vi "capex profile.vi"() -> ()   [LabVIEW 2013]
panel:
  out "Current time":timestamp format="%<%X\n%x>T"
  out "Profile line":dbl
  in  "Stop Profile":bool
  out "profile times":timestamp[](array[timestamp])
  out "profile big chamber temp":dbl[](array[numeric]) format="%.2f"
  out "profile big chamber ramp":dbl[](array[numeric]) format="%.2f"
  out "profile chiller speed":string[](array[string])
  out "profile relay 4":string[](array[string])
  out "profile relay 3":string[](array[string])
  out "profile relay 2":string[](array[string])
  out "profile relay 1":string[](array[string])
  out "profile elapsed time":dbl[](array[numeric]) format="%.2f"
  out "profile AC volts":dbl[](array[numeric]) format="%.2f"
  out "profile AC current limit":dbl[](array[numeric]) format="%.2f"
  out "profile DC volts":dbl[](array[numeric]) format="%.2f"
  out "profile DC current limit":dbl[](array[numeric]) format="%.2f"
  out "profile little chamber temp":dbl[](array[numeric]) format="%.2f"
  out "profile little chamber ramp":dbl[](array[numeric]) format="%.2f"
  out "profile chiller temp":dbl[](array[numeric]) format="%.2f"
  in  "stop":bool
  in  "operation (0:open)":T1(ring)=enum."open or create"
  in  "make template":bool
  out "Profile running":bool
  out "Start time of last executed profile":timestamp
  out "Profile last executed":path
  in  "Loop profile when complete":bool
  in  "Execute profile":bool
  in  "Start in the future":bool
  out "Loaded profile":cluster{timestamp[], dbl[]}[](graph)
  in  "Load Profile":path
  in  "Scheduled start time":timestamp
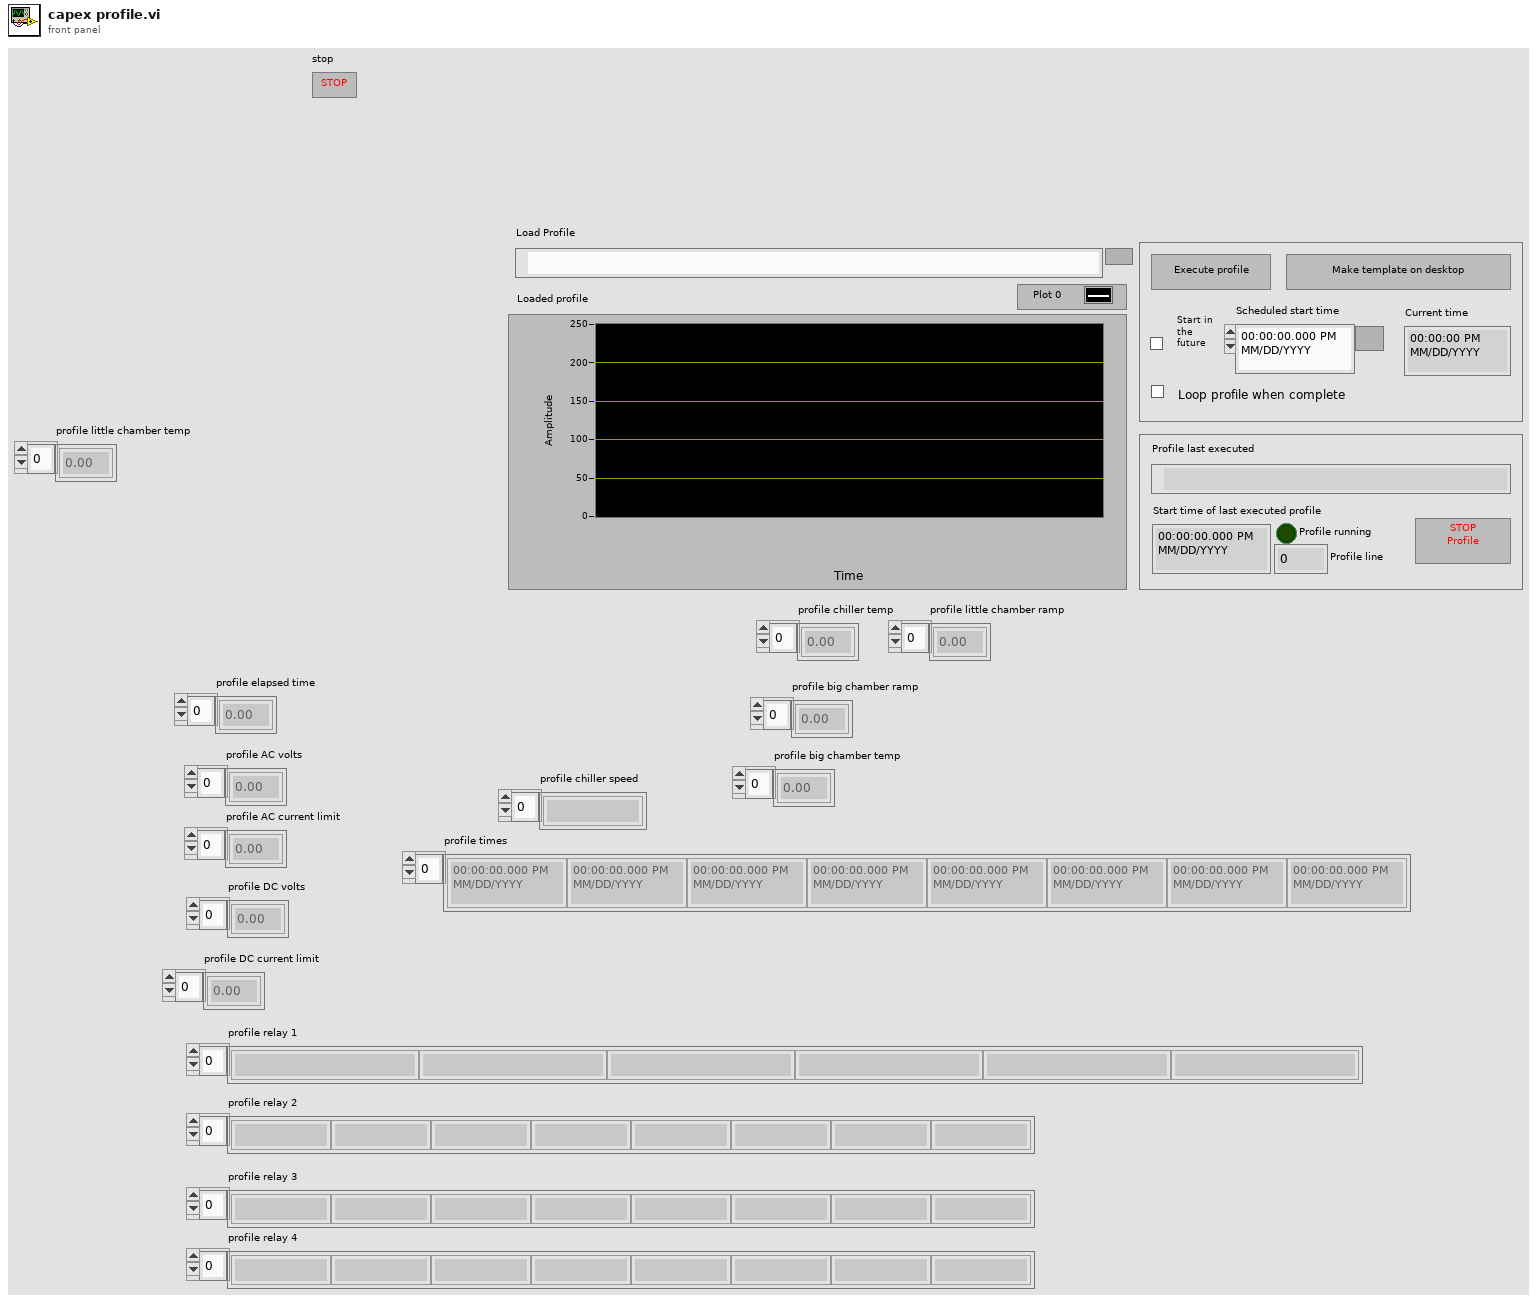
[diagram p1: front panel]
types:
  T1 = enum16{"open", "replace", "create", "open or create", "replace or create", "replace or create with confirmation"}
  T2 = enum8{"Enabled", "Disabled", "Disabled and Grayed Out"}
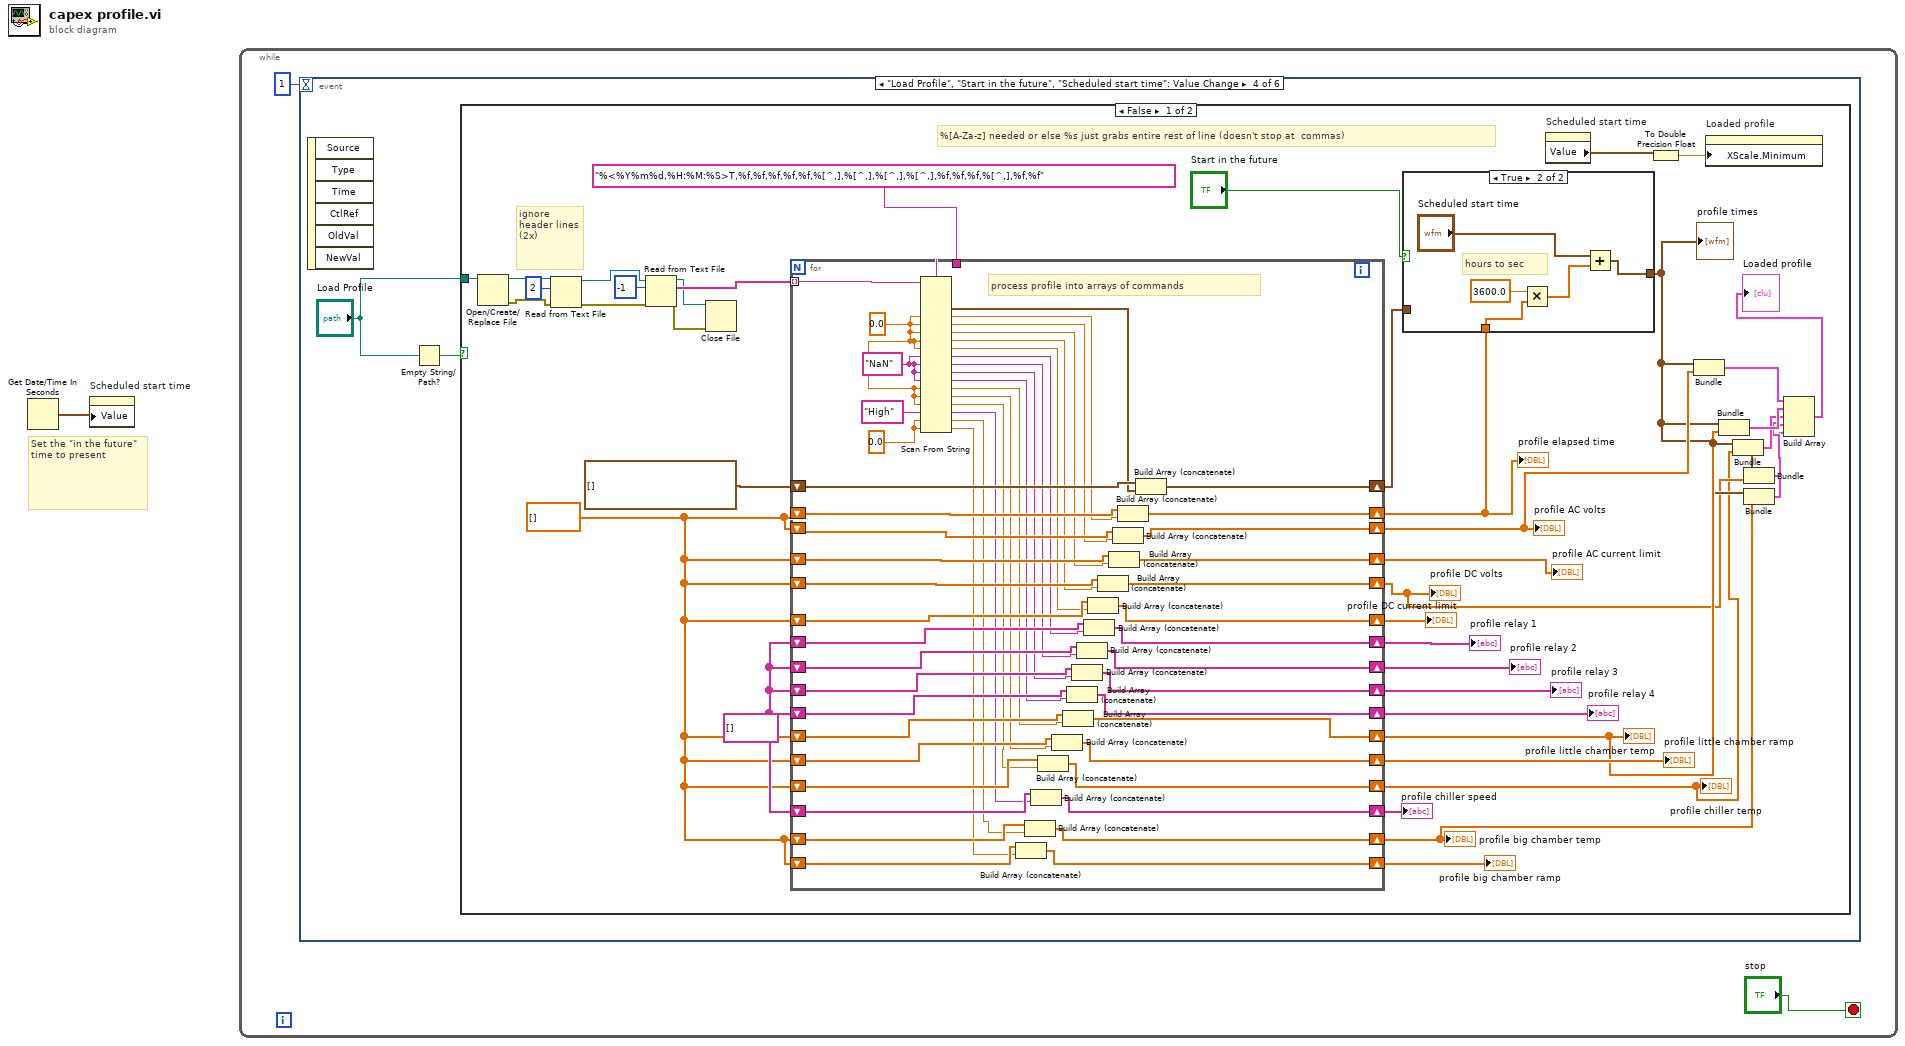
[diagram p0: block diagram]
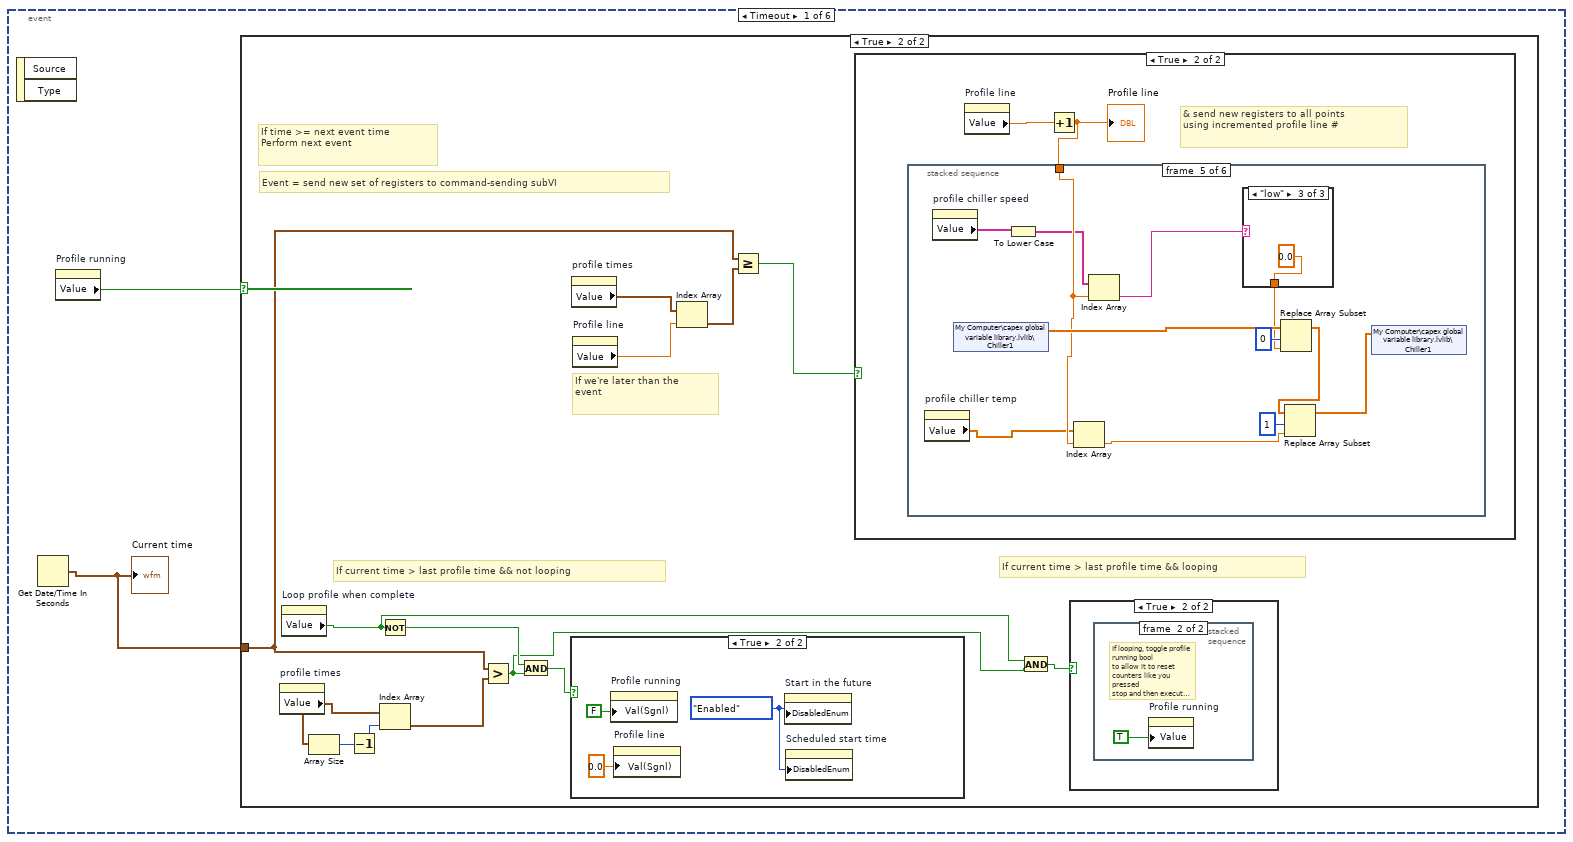
[diagram p2: hidden frame]
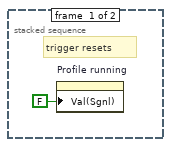
[diagram p5: hidden frame]
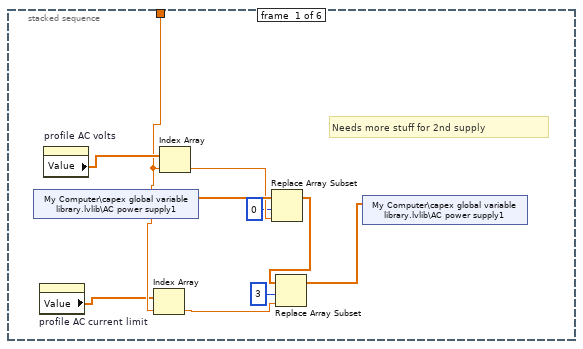
[diagram p7: hidden frame]
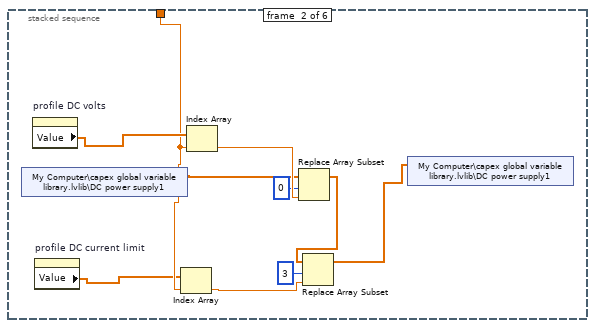
[diagram p8: hidden frame]
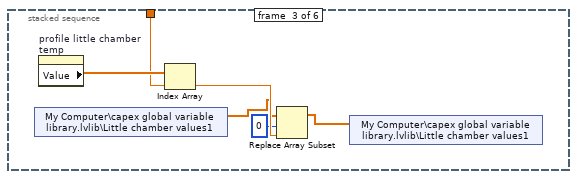
[diagram p9: hidden frame]
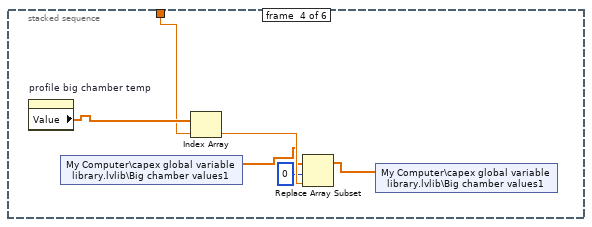
[diagram p10: hidden frame]
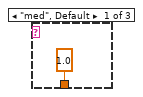
[diagram p11: hidden frame]
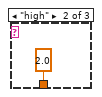
[diagram p12: hidden frame]
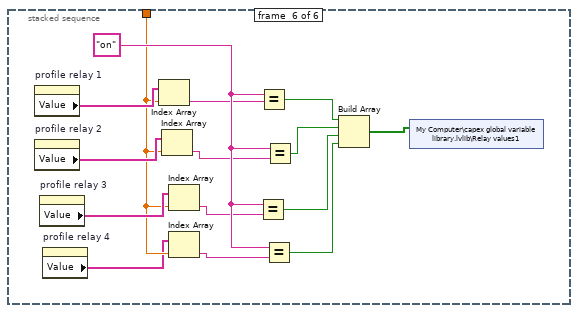
[diagram p13: hidden frame]
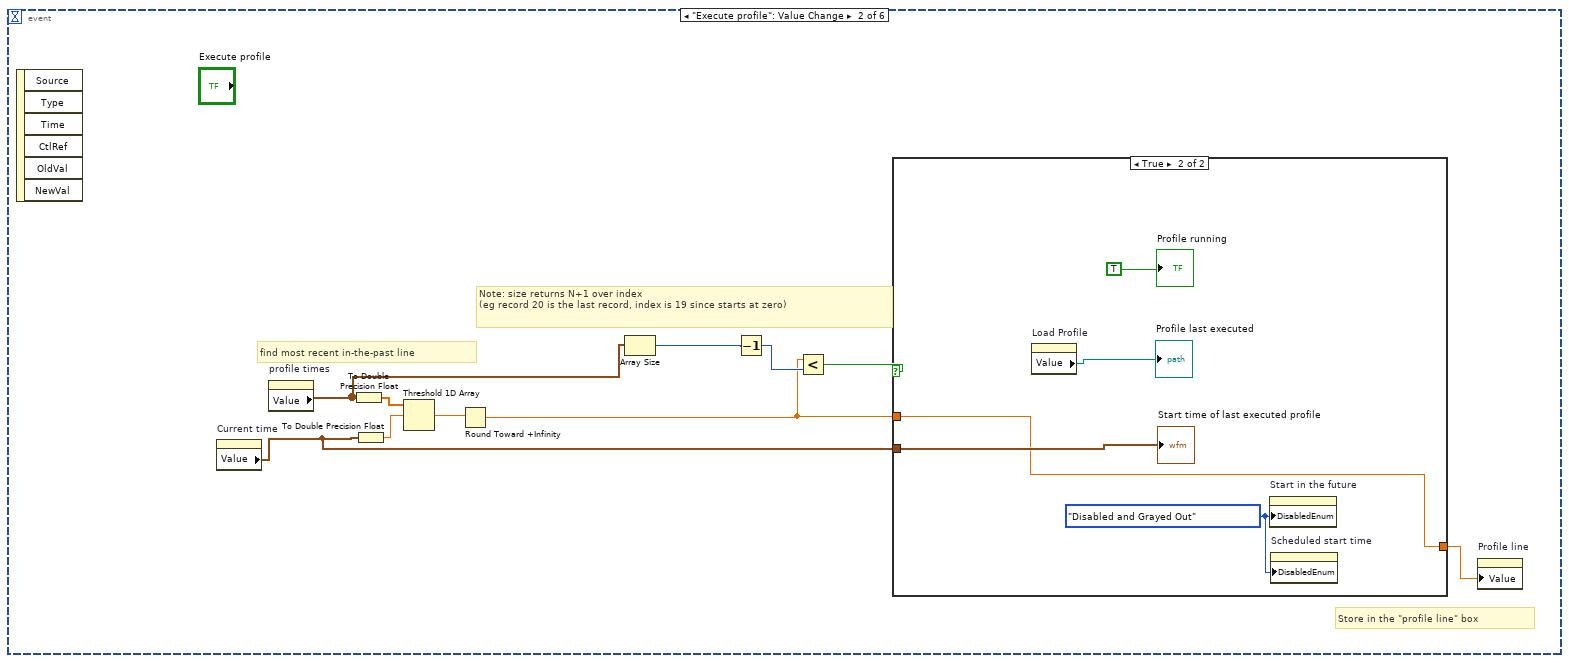
[diagram p15: hidden frame]
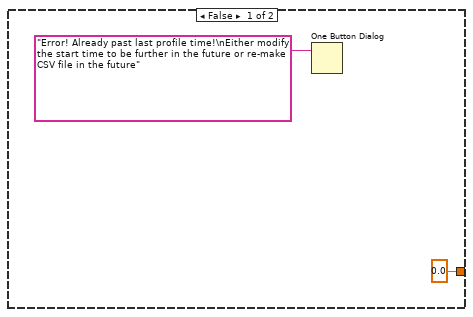
[diagram p16: hidden frame]
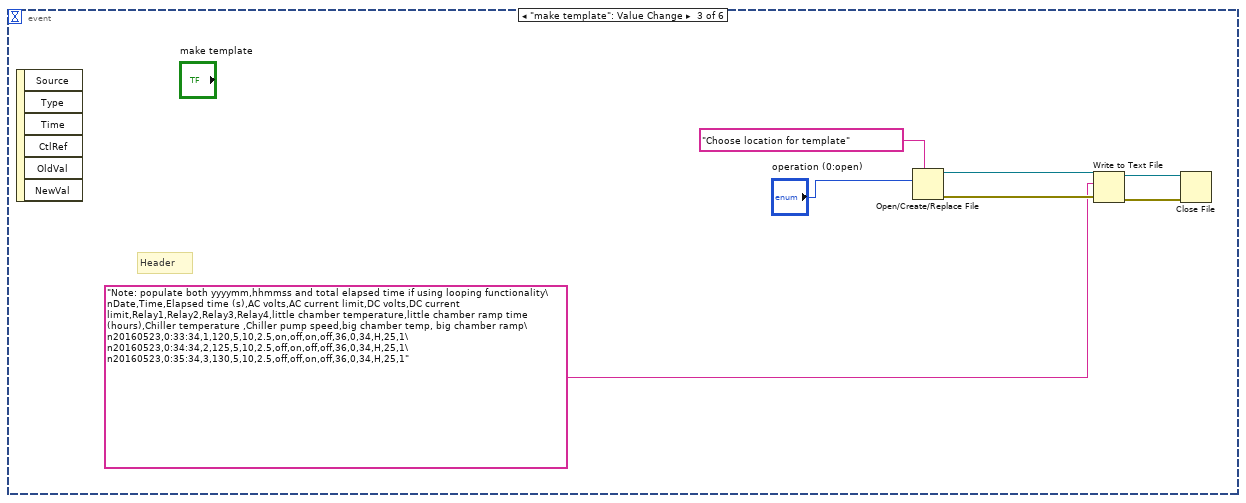
[diagram p17: hidden frame]
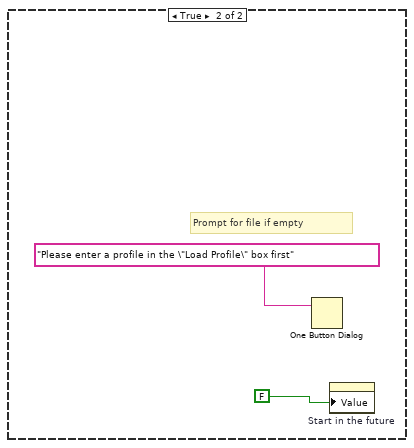
[diagram p19: hidden frame]
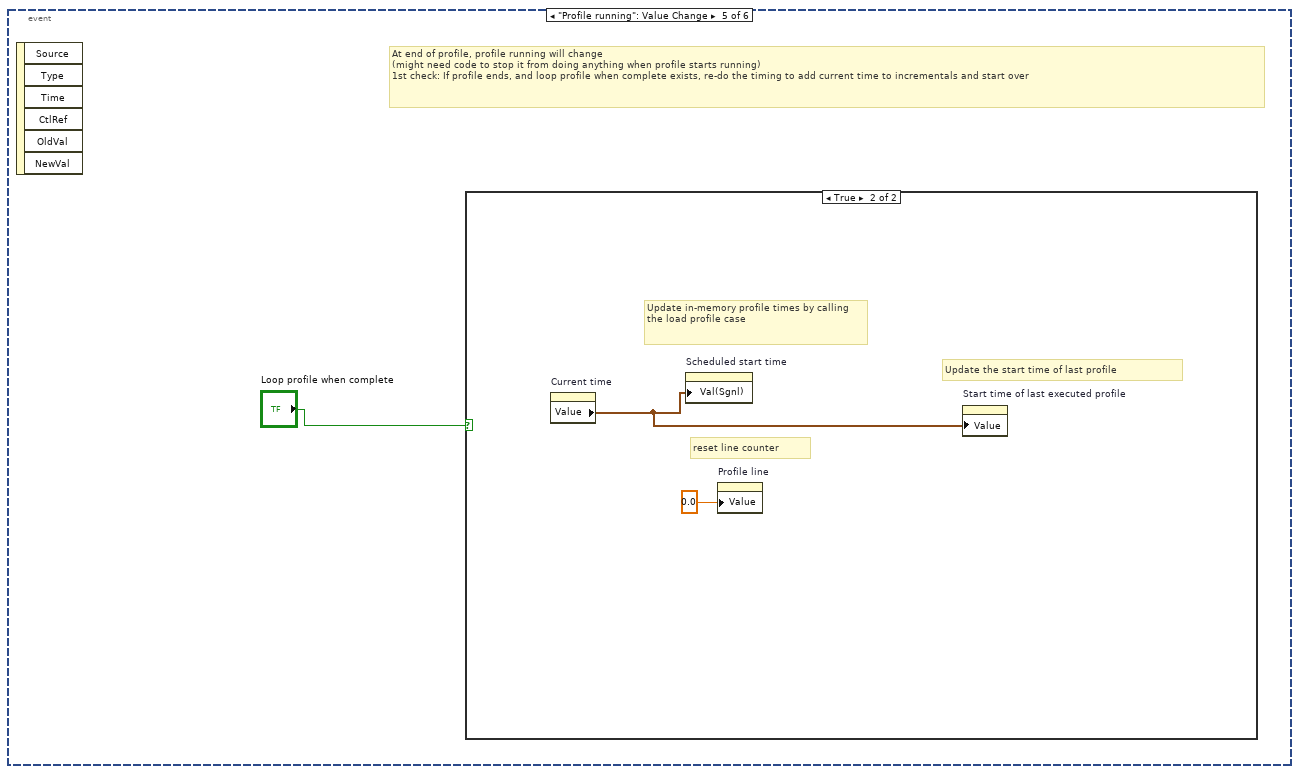
[diagram p20: hidden frame]
diagram:
  # "Set the \"in the future\" time to present"
  n1 = Get Date/Time In Seconds() -> (seconds since 1Jan1904=w1:timestamp)
  n2 = property on="Scheduled start time" class="AbsTime (strict)"("Value"=w1) -> ()  [unwired: 2 in, 2 out]
  n3 = while {
    stop <- "stop" stop-if-true
    n4 = event shown="[3] \"Load Profile\", \"Start in the future\", \"Scheduled start time\": Value Change" {
      selector: _ -> [_ _ _ _ _ _]
      dyn-events: _ -> [_ _ _ _ _ _]
      timeout: 1 -> [_ _ _ _ _ _]
      event Timeout {
        n5 = event-data() -> ()  [unwired: 1 in, 2 out]
        n6 = Get Date/Time In Seconds() -> (seconds since 1Jan1904=w4:timestamp)
        "Current time" <- w4
        n7 = property on="Profile running" class="Bool (strict)"() -> ("Value"=w5:bool)  [unwired: 2 in, 2 out]
        n8 = case shown="True" w5 {
          tunnel: w4 -> [_ w6]
          frame False {
          }
          frame True {
            # "If current time > last profile time && looping"
            # "If we're later than the\nevent"
            # "If current time > last profile time && not looping"
            # "Event = send new set of registers to command-sending subVI"
            # "If time >= next event time\nPerform next event"
            n9 = property on="profile times" class="Arr (strict)"() -> ("Value"=w17:timestamp[])  [unwired: 2 in, 2 out]
            n10 = property on="Loop profile when complete" class="Bool (strict)"() -> ("Value"=w8:bool)  [unwired: 2 in, 2 out]
            n11 = Array Size(array=w17) -> (size(s)=w19:i32)
            n12 = Decrement(x=w19) -> (x-1=w18:i32)
            n13 = Not(x=w8) -> (.not. x?=w14:bool)
            n14 = Index Array(array=w17, index=w18) -> (element=w16:timestamp)
            n15 = Greater?(x=w6, y=w16) -> (0:w7:bool)
            n16 = And(x=w14, y=w7) -> (x .and. y?=w15:bool)
            n17 = case shown="True" w15 {
              frame False {
              }
              frame True {
                w86 = T2."Enabled" ("Disabled")
                n18 = property on="Profile running" class="Bool (strict)"("Val(Sgnl)"=FALSE ("Value (Signaling)")) -> ()  [unwired: 2 in, 2 out]
                n19 = property on="Profile line" class="DigNum (strict)"("Val(Sgnl)"=0.0 ("Value (Signaling)")) -> ()  [unwired: 2 in, 2 out]
                n20 = property on="Start in the future" class="Bool (strict)"("DisabledEnum"=w86) -> ()  [unwired: 2 in, 2 out]
                n21 = property on="Scheduled start time" class="AbsTime (strict)"("DisabledEnum"=w86) -> ()  [unwired: 2 in, 2 out]
              }
            }
            n22 = property on="profile times" class="Arr (strict)"() -> ("Value"=w13:timestamp[])  [unwired: 2 in, 2 out]
            n23 = property on="Profile line" class="DigNum (strict)"() -> ("Value"=w12:dbl)  [unwired: 2 in, 2 out]
            n24 = Index Array(array=w13, index=w12) -> (element=w11:timestamp)
            n25 = Greater Or Equal?(x=w6, y=w11) -> (x >= y?=w10:bool)
            n26 = case shown="True" w10 {
              frame False {
              }
              frame True {
                # "& send new registers to all points\nusing incremented profile line #"
                n27 = property on="Profile line" class="DigNum (strict)"() -> ("Value"=w23:dbl)  [unwired: 2 in, 2 out]
                n28 = Increment(x=w23) -> (x+1=w22:dbl)
                "Profile line" <- w22
                n29 = stacked-sequence {
                  tunnel: w22 -> [w29 w35 w46 w50 w61 w76]
                  frame #0 {
                    # "Needs more stuff for 2nd supply"
                    n30 = shared-variable "My Computer\\capex global variable library.lvlib\\AC power supply1"() -> (w33:dbl[])  [unwired: 1 in, 1 out]
                    n31 = property on="profile AC current limit" class="Arr (strict)"() -> ("Value"=w28:dbl[])  [unwired: 2 in, 2 out]
                    n32 = property on="profile AC volts" class="Arr (strict)"() -> ("Value"=w32:dbl[])  [unwired: 2 in, 2 out]
                    n33 = Index Array(array=w28, index=w29) -> (element=w25:dbl)
                    n34 = Index Array(array=w32, index=w29) -> (element=w31:dbl)
                    n35 = Replace Array Subset(array=w33, new element=w31, index=0) -> (w27:dbl[])
                    n36 = Replace Array Subset(array=w27, new element=w25, index=3) -> (w24:dbl[])
                    n37 = shared-variable "My Computer\\capex global variable library.lvlib\\AC power supply1"(w24) -> ()  [unwired: 1 in, 1 out]
                  }
                  frame #1 {
                    n38 = shared-variable "My Computer\\capex global variable library.lvlib\\DC power supply1"() -> (w37:dbl[])  [unwired: 1 in, 1 out]
                    n39 = property on="profile DC volts" class="Arr (strict)"() -> ("Value"=w36:dbl[])  [unwired: 2 in, 2 out]
                    n40 = property on="profile DC current limit" class="Arr (strict)"() -> ("Value"=w34:dbl[])  [unwired: 2 in, 2 out]
                    n41 = Index Array(array=w34, index=w35) -> (element=w39:dbl)
                    n42 = Index Array(array=w36, index=w35) -> (element=w43:dbl)
                    n43 = Replace Array Subset(array=w37, new element=w43, index=0) -> (w41:dbl[])
                    n44 = Replace Array Subset(array=w41, new element=w39, index=3) -> (w38:dbl[])
                    n45 = shared-variable "My Computer\\capex global variable library.lvlib\\DC power supply1"(w38) -> ()  [unwired: 1 in, 1 out]
                  }
                  frame #2 {
                    n46 = shared-variable "My Computer\\capex global variable library.lvlib\\Little chamber values1"() -> (w45:dbl[])  [unwired: 1 in, 1 out]
                    n47 = property on="profile little chamber temp" class="Arr (strict)"() -> ("Value"=w47:dbl[])  [unwired: 2 in, 2 out]
                    n48 = Index Array(array=w47, index=w46) -> (element=w49:dbl)
                    n49 = Replace Array Subset(array=w45, new element=w49, index=0) -> (w44:dbl[])
                    n50 = shared-variable "My Computer\\capex global variable library.lvlib\\Little chamber values1"(w44) -> ()  [unwired: 1 in, 1 out]
                  }
                  frame #3 {
                    n51 = property on="profile big chamber temp" class="Arr (strict)"() -> ("Value"=w51:dbl[])  [unwired: 2 in, 2 out]
                    n52 = shared-variable "My Computer\\capex global variable library.lvlib\\Big chamber values1"() -> (w53:dbl[])  [unwired: 1 in, 1 out]
                    n53 = Index Array(array=w51, index=w50) -> (element=w55:dbl)
                    n54 = Replace Array Subset(array=w53, new element=w55, index=0) -> (w52:dbl[])
                    n55 = shared-variable "My Computer\\capex global variable library.lvlib\\Big chamber values1"(w52) -> ()  [unwired: 1 in, 1 out]
                  }
                  frame #4 {
                    n56 = property on="profile chiller temp" class="Arr (strict)"() -> ("Value"=w60:dbl[])  [unwired: 2 in, 2 out]
                    n57 = property on="profile chiller speed" class="Arr (strict)"() -> ("Value"=w57:string[])  [unwired: 2 in, 2 out]
                    n58 = shared-variable "My Computer\\capex global variable library.lvlib\\Chiller1"() -> (w67:dbl[])  [unwired: 1 in, 1 out]
                    n59 = To Lower Case(string=w57) -> (all lower case string=w56:string[])
                    n60 = Index Array(array=w60, index=w61) -> (element=w63:dbl)
                    n61 = Index Array(array=w56, index=w61) -> (element=w58:string)
                    n62 = case shown="\"low\"" w58 {
                      tunnel: [1.0 2.0 0.0] -> w59
                      frame "med", Default {
                      }
                      frame "high" {
                      }
                      frame "low" {
                      }
                    }
                    n63 = Replace Array Subset(array=w67, new element=w59, index=0) -> (w65:dbl[])
                    n64 = Replace Array Subset(array=w65, new element=w63, index=1) -> (w62:dbl[])
                    n65 = shared-variable "My Computer\\capex global variable library.lvlib\\Chiller1"(w62) -> ()  [unwired: 1 in, 1 out]
                  }
                  frame #5 {
                    w85 = "on"
                    n66 = property on="profile relay 1" class="Arr (strict)"() -> ("Value"=w77:string[])  [unwired: 2 in, 2 out]
                    n67 = property on="profile relay 2" class="Arr (strict)"() -> ("Value"=w78:string[])  [unwired: 2 in, 2 out]
                    n68 = property on="profile relay 3" class="Arr (strict)"() -> ("Value"=w79:string[])  [unwired: 2 in, 2 out]
                    n69 = property on="profile relay 4" class="Arr (strict)"() -> ("Value"=w75:string[])  [unwired: 2 in, 2 out]
                    n70 = Index Array(array=w77, index=w76) -> (element=w71:string)
                    n71 = Index Array(array=w78, index=w76) -> (element=w72:string)
                    n72 = Index Array(array=w79, index=w76) -> (element=w73:string)
                    n73 = Index Array(array=w75, index=w76) -> (element=w74:string)
                    n74 = Equal?(x=w85, y=w73) -> (x = y?=w83:bool)
                    n75 = Equal?(x=w85, y=w71) -> (x = y?=w81:bool)
                    n76 = Equal?(x=w85, y=w74) -> (x = y?=w84:bool)
                    n77 = Equal?(x=w85, y=w72) -> (x = y?=w82:bool)
                    n78 = Build Array(w81, w82, w83, w84) -> (w80:bool[])
                    n79 = shared-variable "My Computer\\capex global variable library.lvlib\\Relay values1"(w80) -> ()  [unwired: 1 in, 1 out]
                  }
                }
              }
            }
            n80 = And(x=w8, y=w7) -> (x .and. y?=w9:bool)
            n81 = case shown="True" w9 {
              frame False {
              }
              frame True {
                n82 = stacked-sequence {
                  frame #0 {
                    # "trigger resets"
                    n83 = property on="Profile running" class="Bool (strict)"("Val(Sgnl)"=FALSE ("Value (Signaling)")) -> ()  [unwired: 2 in, 2 out]
                  }
                  frame #1 {
                    # "If looping, toggle profile running bool\nto allow it to reset counters like you pressed\nstop and then execute again"
                    n84 = property on="Profile running" class="Bool (strict)"("Value"=TRUE ("Value (Signaling)")) -> ()  [unwired: 2 in, 2 out]
                  }
                }
              }
            }
          }
        }
      }
      event "Execute profile": Value Change {
        # "Note: size returns N+1 over index\n(eg record 20 is the last record, index is 19 since starts at zero)"
        # "Store in the \"profile line\" box"
        # "find most recent in-the-past line"
        n85 = event-data() -> ()  [unwired: 1 in, 6 out]
        n86 = property on="Current time" class="AbsTime (strict)"() -> ("Value"=w89:timestamp)  [unwired: 2 in, 2 out]
        n87 = property on="profile times" class="Arr (strict)"() -> ("Value"=w96:timestamp[])  [unwired: 2 in, 2 out]
        n88 = To Double Precision Float(number=w96) -> (double precision float=w97:dbl[])
        n89 = To Double Precision Float(number=w89) -> (double precision float=w98:dbl)
        n90 = Threshold 1D Array(2:w98, 3:w97) -> (0:w94:dbl)  [unwired: 1 in]
        n91 = Round Toward +Infinity(x=w94) -> (ceil(x): smallest int >= x=w90:dbl)
        n92 = Array Size(array=w96) -> (size(s)=w93:i32)
        n93 = Decrement(x=w93) -> (x-1=w92:i32)
        n94 = Less?(x=w90, y=w92) -> (x < y?=w95:bool)
        n95 = case shown="True" w95 {
          tunnel: [0.0 w101] -> w91
          tunnel: w90 -> [_ w101]
          tunnel: w89 -> [_ w103]
          frame False {
            n96 = One Button Dialog(message="Error! Already past last profile time!\nEither modify the start time to be further in the future or re-make CSV file in the future") -> ()  [unwired: 1 in, 1 out]
          }
          frame True {
            w102 = T2."Disabled and Grayed Out" ("Disabled")
            n97 = property on="Load Profile" class="Path"() -> ("Value"=→"Profile last executed":path)  [unwired: 2 in, 2 out]
            n98 = property on="Start in the future" class="Bool (strict)"("DisabledEnum"=w102) -> ()  [unwired: 2 in, 2 out]
            n99 = property on="Scheduled start time" class="AbsTime (strict)"("DisabledEnum"=w102) -> ()  [unwired: 2 in, 2 out]
            "Profile running" <- TRUE
            "Start time of last executed profile" <- w103
          }
        }
        n100 = property on="Profile line" class="DigNum (strict)"("Value"=w91) -> ()  [unwired: 2 in, 2 out]
      }
      event "make template": Value Change {
        # "Header"
        n101 = event-data() -> ()  [unwired: 1 in, 6 out]
        n102 = Open/Create/Replace File(prompt="Choose location for template", operation (0:open)="operation (0:open)") -> (refnum out=w111:refnum<file>, error out=w108:errorcluster)  [unwired: 4 in, 1 out]
        n103 = Write to Text File(file (use dialog)=w111, text="Note: populate both yyyymm,hhmmss and total elapsed time if using looping functionality\nDate,Time,Elapsed time (s),AC volts,AC current limit,DC volts,DC current limit,Relay1,Relay2,Relay3,Relay4,little chamber temperature,little chamber ramp time (hours),Chiller temperature ,Chiller pump speed,big chamber temp, big chamber ramp\n20160523,0:33:34,1,120,5,10,2.5,on,off,on,off,36,0,34,H,25,1\n20160523,0:34:34,2,125,5,10,2.5,off,on,off,off,36,0,34,H,25,1\n20160523,0:35:34,3,130,5,10,2.5,off,off,on,off,36,0,34,H,25,1", error in=w108) -> (refnum out=w110:refnum<file>, error out=w109:errorcluster)  [unwired: 1 in, 1 out]
        n104 = Close File(refnum=w110, error in=w109) -> ()  [unwired: 2 out]
      }
      event "Load Profile", "Start in the future", "Scheduled start time": Value Change {
        n105 = event-data() -> ()  [unwired: 1 in, 6 out]
        n106 = Empty String/Path?(string/path="Load Profile") -> (empty?=w113:bool)
        n107 = case shown="False" w113 {
          tunnel: "Load Profile" -> [w123 _]
          frame False {
            w135 = string[] []
            w134 = dbl[] []
            # "ignore header lines (2x)"
            # "%[A-Za-z] needed or else %s just grabs entire rest of line (doesn't stop at  commas)"
            n108 = Open/Create/Replace File(file path (use dialog)=w123) -> (refnum out=w139:refnum<file>, error out=w141:errorcluster)  [unwired: 5 in, 1 out]
            n109 = Read from Text File(file (use dialog)=w139, count=2, error in=w141) -> (refnum out=w138:refnum<file>, error out=w140:errorcluster)  [unwired: 1 in, 2 out]
            n110 = Read from Text File(file (use dialog)=w138, count=-1, error in=w140) -> (refnum out=w143:refnum<file>, text=w144:string[], error out=w142:errorcluster)  [unwired: 1 in, 1 out]
            n111 = Close File(refnum=w143, error in=w142) -> ()  [unwired: 2 out]
            n112 = for {
              tunnel: "%<%Y%m%d,%H:%M:%S>T,%f,%f,%f,%f,%f,%[^,],%[^,],%[^,],%[^,],%f,%f,%f,%[^,],%f,%f" ("format string") -> [w214]
              shift-right: [w212] -> w131
              shift-left: w134 -> [w191]
              shift-right: [w211] -> w129
              shift-left: w134 -> [w189]
              shift-right: [w210] -> w152
              shift-left: w134 -> [w187]
              shift-right: [w209] -> w126
              shift-left: w134 -> [w185]
              shift-right: [w208] -> w151
              shift-left: w134 -> [w183]
              shift-right: [w207] -> w150
              shift-left: w135 -> [w181]
              shift-right: [w206] -> w149
              shift-left: w135 -> [w179]
              shift-right: [w205] -> w148
              shift-left: w135 -> [w177]
              shift-right: [w204] -> w147
              shift-left: w135 -> [w175]
              shift-right: [w203] -> w128
              shift-left: w134 -> [w173]
              shift-right: [w202] -> w130
              shift-left: w134 -> [w171]
              shift-right: [w201] -> w125
              shift-left: w134 -> [w169]
              shift-right: [w200] -> w146
              shift-left: w135 -> [w167]
              shift-right: [w197] -> w124
              shift-left: w134 -> [w165]
              shift-right: [w196] -> w145
              shift-left: w134 -> [w163]
              shift-right: [w195] -> w132
              shift-left: timestamp[] [] -> [w193]
              tunnel: w144 -> [w161] mode=indexing
              w194 = 0.0 ("default value 15")
              w199 = "NaN" ("default value 15")
              w198 = 0.0
              # "process profile into arrays of commands"
              n113 = Scan From String(format string=w214, input string=w161, default 2=w198, default 3=w198, default 4=w198, default 5=w198, default 6=w198, default 7=w199, default 8=w199, default 9=w199, default 10=w199, default 11=w198, default 12=w198, default 13=w198, default 14="High" ("default value 19"), default 15=w194, default 16=w194) -> (output 1=w192:timestamp, output 2=w190:dbl, output 3=w188:dbl, output 4=w186:dbl, output 5=w184:dbl, output 6=w182:dbl, output 7=w180:string, output 8=w178:string, output 9=w176:string, output 10=w174:string, output 11=w172:dbl, output 12=w170:dbl, output 13=w168:dbl, output 14=w166:string, output 15=w164:dbl, output 16=w162:dbl)  [unwired: 3 in, 3 out]
              n114 = Build Array (concatenate)(w163, w162) -> (w196:dbl[])
              n115 = Build Array (concatenate)(w165, w164) -> (w197:dbl[])
              n116 = Build Array (concatenate)(w167, w166) -> (w200:string[])
              n117 = Build Array (concatenate)(w169, w168) -> (w201:dbl[])
              n118 = Build Array (concatenate)(w171, w170) -> (w202:dbl[])
              n119 = Build Array (concatenate)(w173, w172) -> (w203:dbl[])
              n120 = Build Array (concatenate)(w175, w174) -> (w204:string[])
              n121 = Build Array (concatenate)(w177, w176) -> (w205:string[])
              n122 = Build Array (concatenate)(w179, w178) -> (w206:string[])
              n123 = Build Array (concatenate)(w181, w180) -> (w207:string[])
              n124 = Build Array (concatenate)(w183, w182) -> (w208:dbl[])
              n125 = Build Array (concatenate)(w185, w184) -> (w209:dbl[])
              n126 = Build Array (concatenate)(w187, w186) -> (w210:dbl[])
              n127 = Build Array (concatenate)(w189, w188) -> (w211:dbl[])
              n128 = Build Array (concatenate)(w191, w190) -> (w212:dbl[])
              n129 = Build Array (concatenate)(w193, w192) -> (w195:timestamp[])
            }
            "profile chiller temp" <- w125
            "profile little chamber ramp" <- w130
            "profile little chamber temp" <- w128
            "profile DC current limit" <- w151
            "profile DC volts" <- w126
            "profile AC current limit" <- w152
            "profile AC volts" <- w129
            "profile elapsed time" <- w131
            "profile relay 1" <- w150
            "profile relay 2" <- w149
            "profile relay 3" <- w148
            "profile relay 4" <- w147
            "profile chiller speed" <- w146
            "profile big chamber ramp" <- w145
            "profile big chamber temp" <- w124
            n130 = case shown="True" "Start in the future" {
              tunnel: [w155 w160] -> w127
              tunnel: w132 -> [w155 _]
              tunnel: w131 -> [_ w157]
              frame False {
              }
              frame True {
                # "hours to sec"
                n131 = Multiply(x=3600.0, y=w157) -> (x*y=w158:dbl[])
                n132 = Add(x="Scheduled start time", y=w158) -> (x+y=w160:timestamp[])
              }
            }
            "profile times" <- w127
            n133 = property on="Scheduled start time" class="AbsTime (strict)"() -> ("Value"=w115:timestamp)  [unwired: 2 in, 2 out]
            n134 = To Double Precision Float(number=w115) -> (double precision float=w116:dbl)
            n135 = Bundle(w127, w129) -> (w122:cluster{timestamp[], dbl[]})  [unwired: 1 in]
            n136 = property on="Loaded profile" class="XYGraph (strict)"("XScale.Minimum"=w116) -> ()  [unwired: 2 in, 2 out]
            n137 = Bundle(w127, w128) -> (w121:cluster{timestamp[], dbl[]})  [unwired: 1 in]
            n138 = Bundle(w127, w125) -> (w120:cluster{timestamp[], dbl[]})  [unwired: 1 in]
            n139 = Bundle(w127, w126) -> (w119:cluster{timestamp[], dbl[]})  [unwired: 1 in]
            n140 = Bundle(w127, w124) -> (w118:cluster{timestamp[], dbl[]})  [unwired: 1 in]
            n141 = Build Array(w122, w121, w120, w119, w118) -> (→"Loaded profile":cluster{timestamp[], dbl[]}[])
          }
          frame True {
            # "Prompt for file if empty"
            n142 = One Button Dialog(message="Please enter a profile in the \"Load Profile\" box first") -> ()  [unwired: 1 in, 1 out]
            n143 = property on="Start in the future" class="Bool (strict)"("Value"=FALSE ("Value (Signaling)")) -> ()  [unwired: 2 in, 2 out]
          }
        }
      }
      event "Profile running": Value Change {
        # "At end of profile, profile running will change\n(might need code to stop it from doing anything when profile starts running)\n1st check: If profile ends, and loop profile when complete exists, re-do the timing to add current time to incrementals and start over"
        n144 = event-data() -> ()  [unwired: 1 in, 6 out]
        n145 = case shown="True" "Loop profile when complete" {
          frame False {
          }
          frame True {
            # "Update the start time of last profile"
            # "Update in-memory profile times by calling the load profile case"
            # "reset line counter"
            n146 = property on="Current time" class="AbsTime (strict)"() -> ("Value"=w219:timestamp)  [unwired: 2 in, 2 out]
            n147 = property on="Scheduled start time" class="AbsTime (strict)"("Val(Sgnl)"=w219) -> ()  [unwired: 2 in, 2 out]
            n148 = property on="Profile line" class="DigNum (strict)"("Value"=0.0 ("Value (Signaling)")) -> ()  [unwired: 2 in, 2 out]
            n149 = property on="Start time of last executed profile" class="AbsTime (strict)"("Value"=w219) -> ()  [unwired: 2 in, 2 out]
          }
        }
      }
      event "Stop Profile": Value Change {
        w220 = T2."Enabled" ("Disabled")
        n150 = event-data() -> ()  [unwired: 1 in, 6 out]
        n151 = property on="Start in the future" class="Bool (strict)"("DisabledEnum"=w220) -> ()  [unwired: 2 in, 2 out]
        n152 = property on="Profile running" class="Bool (strict)"("Val(Sgnl)"=FALSE ("Value (Signaling)")) -> ()  [unwired: 2 in, 2 out]
        n153 = property on="Loop profile when complete" class="Bool (strict)"("Val(Sgnl)"=FALSE ("Value (Signaling)")) -> ()  [unwired: 2 in, 2 out]
        n154 = property on="Scheduled start time" class="AbsTime (strict)"("DisabledEnum"=w220) -> ()  [unwired: 2 in, 2 out]
      }
    }
  }
